vi "Solve Linear Equations (single right hand).vi"(2 "matrix type":T1, 3 "Known Vector":dbl[](array[numeric]) format="%.2f", 4 "Input Matrix":T2) -> (0 "error":i32, 1 "Solution Vector":dbl[](array[numeric]) format="%.2f")   [LabVIEW 2014, in "NI_AALPro.lvlib"]
doc: "Solves a linear system AX = Y. The data types you wire to the <B>Input Matrix</B> and <B>Known Vector</B> inputs determine the polymorphic instance to use."
uses:
  NI_AALPro.lvlib
  RealMatrix.ctl
  Matrix Type of Inverse Matrix.ctl
  Solve Linear Eqs (Gen, single right hand).vi
  NI_AALBase.lvlib
  NI_Matrix.lvlib
panel:
  # "Solve Linear Equations"
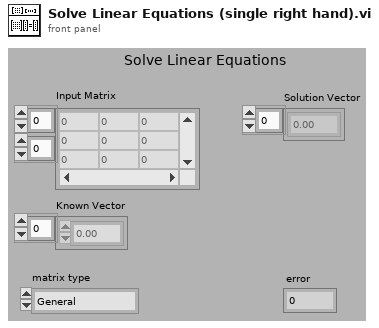
[diagram p1: front panel]
types:
  T1 = typedef "NI_AALBase.lvlib/Matrix Type of Inverse Matrix.ctl" = enum32{"General", "Positive Definite", "Lower Triangular", "Upper Triangular"}
  T2 = typedef "NI_Matrix.lvlib/RealMatrix.ctl" = dbl[][]
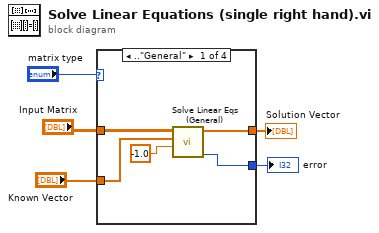
[diagram p0: block diagram]
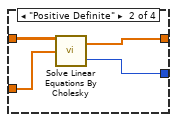
[diagram p2: hidden frame]
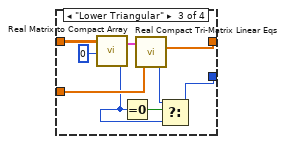
[diagram p3: hidden frame]
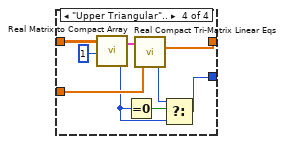
[diagram p4: hidden frame]
diagram:
  n1 = case shown="..\"General\"" "matrix type" {
    tunnel: "Known Vector" -> [w9 w12 w20 w29]
    tunnel: [w7 w11 w15 w24] -> w4
    tunnel: [w8 w14 w19 w28] -> w3
    tunnel: "Input Matrix" -> [w10 w13 w22 w31]
    frame .."General" {
      n2 = call-poly "Solve Linear Eqs (General).vi"("relative tolerance"=-1.0, "Known Vector"=w9, "Input Matrix"=w10) -> ("error"=w7:i32, "Solution Vector"=w8:dbl[])  [unwired: 7 in]
    }
    frame "Positive Definite" {
      n3 = call "Solve Linear Equations By Cholesky.vi"("Known Vector"=w12, "Input Matrix"=w13) -> ("error"=w11:i32, "Solution Vector"=w14:dbl[])  [unwired: 1 in]
    }
    frame "Lower Triangular" {
      n4 = call "Real Matrix to Compact Array.vi"("matrix type"=0, "Matrix A"=w22) -> ("error"=w17:i32, "Compact Array"=w21:cluster{"Compact Array":dbl[], "array type":i32})
      n5 = Equal To 0?(x=w17) -> (x = 0?=w18:bool)
      n6 = call "Real Compact Tri-Matrix Linear Eqs.vi"("Known Vector"=w20, "Triangular Compact Array"=w21) -> ("error"=w16:i32, "Solution Vector"=w19:dbl[])
      n7 = Select(t=w16, s=w18, f=w17) -> (s? t:f=w15:i32)
    }
    frame "Upper Triangular".. {
      n8 = call "Real Matrix to Compact Array.vi"("matrix type"=1, "Matrix A"=w31) -> ("error"=w26:i32, "Compact Array"=w30:cluster{"Compact Array":dbl[], "array type":i32})
      n9 = Equal To 0?(x=w26) -> (x = 0?=w27:bool)
      n10 = call "Real Compact Tri-Matrix Linear Eqs.vi"("Known Vector"=w29, "Triangular Compact Array"=w30) -> ("error"=w25:i32, "Solution Vector"=w28:dbl[])
      n11 = Select(t=w25, s=w27, f=w26) -> (s? t:f=w24:i32)
    }
  }
  "error" <- w4
  "Solution Vector" <- w3
